vi "Save Changes.vi"   [LabVIEW 2014, in "nisyscfg.lvlib"]
doc: "Saves changes made to hardware and systems."
uses:
  nisyscfg.lvlib
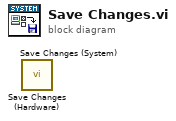
[diagram p0: block diagram]
diagram:
  n1 = call "Save Changes (Hardware).vi"() -> ()  [unwired: 8 in, 4 out]
  n2 = call "Save Changes (System).vi"() -> ()  [unwired: 8 in, 4 out]
